vi "DAQ_E_mIO_DIO.read word.vi"(0 "i ref in":refnum<vi>, 2 "wordIndex":u32, 3 "ms timeout (10000)":i32=10000, 5 "error in (no error)":errorcluster) -> (14 "i ref out":refnum<vi>, 16 "word":u8, 17 "timed out":bool, 19 "error out":errorcluster)   [LabVIEW 2014, in "DAQ_E_mIO_DIO.lvlib"]
doc: "Reads a word from the digital input\n\nLicense Agreement for this software:\n\nCopyright (C)\nGesellschaft für Schwerionenforschung, GSI\nPlanckstr. 1\n64291 Darmstadt\nGermany\n\nContact: D.Beck@gsi.de \n\nThis program is free software; you can redistribute it and/or modify it under the terms of the GNU General Public License as published by the Free Software Foundation; either version 2 of the license, or (at your option) any later version.\n\nThis program is distributed in the hope that it will be useful, but WITHOUT ANY WARRANTY; without even the implied warranty of MERCHANTABILITY or FITNESS FOR A PARTICULAR PURPOSE. See the GNU General License for more details (http://www.gnu.org).\n\nGesellschaft für Schwerionenforschung, GSI\nPlanckstr. 1, 64291 Darmstadt, Germany\nFor all questions and ideas contact: M.Richter@gsi.de, H.Brand@gsi.de or D.Beck@gsi.de.\nLast update: 17-JUN-2004"
uses:
  DAQ_E_mIO_DIO.lvlib
  CS_Core/CSSystem/CoreDefs/CoreDefs.error_type.ctl
  CS_Core/CSApplicationBaseClasses/DigiIOBase/DigiIOBase.directionType.ctl
  CS_Core/CSApplicationBaseClasses/DigiIOBase/DigiIOBase.serviceType.ctl
  CSlibraries/UtilityLib/UtilityLib.valueStatus.ctl
  <vilib>/DAQmx/read.llb/DAQmx Read (Digital 1D Bool 1Chan 1Samp).vi
  CS_Core/CSSystem/CoreLib/CoreLib.lvlib
  CS_Core/CSApplicationBaseClasses/DigiIOBase/DigiIOBase.lvlib
  CSlibraries/UtilityLib/UtilityLib.lvlib
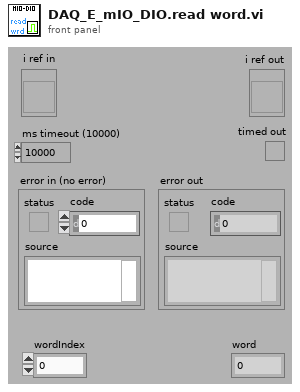
[diagram p1: front panel]
types:
  T1 = typedef "CoreDefs.error_type.ctl" = enum16{"no error", "can't load process", "can't unload process", "process does not exist", "can't install process", "can't remove process", "unknown function", "time out", "can't execute function", "duplicate queue name", "super not found", "caller queue invalid", "can't ping process", "unknown error", "VISA Error", "VISA timeout", "GPIB timeout", "GPIB error", "communication error", "data type mismatch", "can't read data from OPC server", "can't write data to OPC server", "OET error", "function not implemented", "process already exists", "invalid Shared Variable name", "error writing Shared Variable", "error reading Shared Variable", "invalid client name", "corrupt database", "unknown class", "call not authorized", "parameter out of range", "OET timeout: can't get data to modify", "invalid queue name", "requested operation incompatible with current state", "event undefined", "event disabled", "state undefined", "caller is not a friend", "EventBuilder: bad eventID", "EventBuilder: no DAQ devices", "a thread must not stop itself", "UNUSED ELEMENT4", "DiscArchiver: eventData incomplete", "DiscArchiver: eventData does not belong to run", "DiscArchiver: can't open file", "DiscArchiver: can't write to file", "DiscArchiver: available disc space low", "can't acquire semaphore", "error reading data from database", "notifier object is not existing", "can't register process", "can't unregister process", "illegal event type", "object disabled", "object already exists", "can't change state", "Instrument not found", "no connection to remote node", "invalid reference", "N/A", "UNUSED ELEMENT 1", "element not found", "illegal TCP/IP connection detected", "object does not exist", "invalid access ID", "unknown CS system", "invalid privilige", "unsupported data type", "unsupported server type", "IO server already exists", "Shared Variable already exists"}
  T2 = typedef "UtilityLib.lvlib/UtilityLib.valueStatus.ctl" = enum16{"no info available", "stand by/off", "on", "warning", "alarm/malfunction", "not implemented", "user action required", "important information", "system default", "control default", "indicator default", "button default"}
  T3 = typedef "DigiIOBase.lvlib/DigiIOBase.serviceType.ctl" = enum16{"bit", "word"}
  T4 = typedef "DigiIOBase.lvlib/DigiIOBase.directionType.ctl" = enum16{"unknown", "update actual value", "update nominal value", "update both"}
  T5 = typedef "DAQ_E_mIO_DIO.lvlib/DAQ_E_mIO_DIO.i attribute.ctl" = cluster{"DOutChannel":refnum<k21>, "DInChannel":refnum<k21>, "nOfBitsIn":i32, "nOfBitsOut":i32}
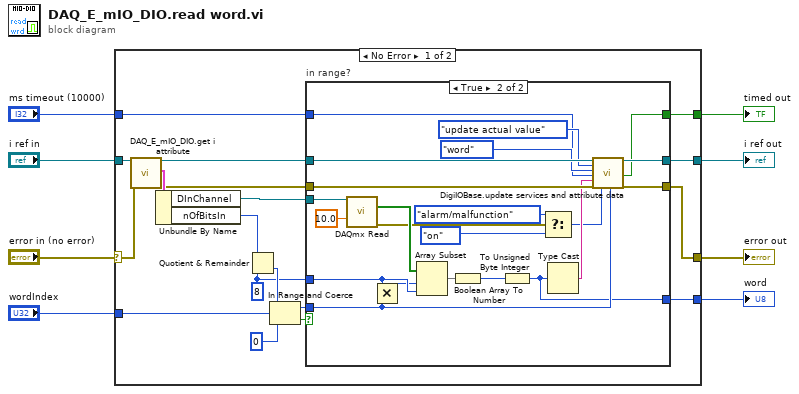
[diagram p0: block diagram]
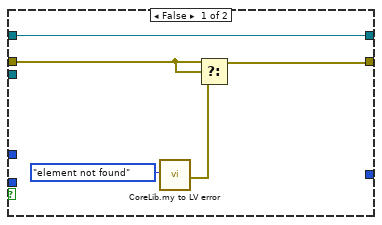
[diagram p2: hidden frame]
diagram:
  n1 = case shown="No Error" "error in (no error)" {
    selector: "error in (no error)" -> [w18 w54]
    tunnel: "i ref in" -> [w19 w55]
    tunnel: [w26 w55] -> w7
    tunnel: [w25 w54] -> w6
    tunnel: "wordIndex" -> [w23 _]
    tunnel: [w20 _] -> w4
    tunnel: "ms timeout (10000)" -> [w13 _]
    tunnel: [w12 _] -> w1
    frame No Error {
      w9 = 8 ("y")
      n2 = call "DAQ_E_mIO_DIO.get i attribute.vi"("i ref in"=w19, "error in (no error)"=w18) -> ("i ref out"=w15:refnum<vi>, "i attribute"=w17:T5, "error out"=w16:errorcluster)  [unwired: 15 in]
      n3 = Unbundle By Name(w17) -> ("DInChannel"=w14:refnum<k21>, "nOfBitsIn"=w11:i32)
      n4 = Quotient & Remainder(x=w11, y=w9) -> (floor(x/y)=w10:i32)  [unwired: 1 out]
      n5 = In Range and Coerce(upper limit=w10, x=w23, lower limit=u32 0) -> (coerced(x)=w22:u32, In Range?=w21:bool)
      n6 = case "in range?" shown="True" w21 {
        tunnel: w15 -> [w31 w50]
        tunnel: w16 -> [w30 w48]
        tunnel: [w31 w49] -> w26
        tunnel: [w29 w47] -> w25
        tunnel: w22 -> [_ w35]
        tunnel: [_ w32] -> w20
        tunnel: w14 -> [_ w52]
        tunnel: w13 -> [_ w44]
        tunnel: [_ w41] -> w12
        tunnel: w9 -> [_ w36]
        frame False {
          n7 = call "CoreLib.my to LV error.vi"("ErrorTypes"=CoreDefs.error_type."element not found") -> ("myErrorCluster"=w28:errorcluster)  [unwired: 17 in, 1 out]
          n8 = Select(t=w30, s=w30, f=w28) -> (s? t:f=w29:errorcluster)
        }
        frame True {
          n9 = call-poly <vilib>:"DAQmx Read.vi"("task/channels in"=w52, "timeout"=10.0) -> ("data"=w51:bool[], "error out"=w40:errorcluster)  [unwired: 11 in, 1 out]
          n10 = Multiply(x=w36, y=w35) -> (x*y=w34:u32)
          n11 = Array Subset(array=w51, index=w34, length=w36) -> (w43:bool[])
          n12 = Boolean Array To Number(Boolean array=w43) -> (number=w33:u32)
          n13 = To Unsigned Byte Integer(number=w33) -> (unsigned 8bit integer=w32:u8)
          n14 = Select(t=UtilityLib.valueStatus."alarm/malfunction", s=w40, f=UtilityLib.valueStatus."on" ("quality")) -> (s? t:f=w37:T2)
          n15 = Type Cast(x=w32) -> (*(type *) &x=w42:string)  [unwired: 1 in]
          n16 = call "DigiIOBase.update services and attribute data.vi"("i ref in"=w50, "direction"=DigiIOBase.directionType."update actual value", "service"=DigiIOBase.serviceType."word", "ms timeout (10000)"=w44, "value"=w42, "error in (no error)"=w48, "quality"=w37, "index"=w35) -> ("i ref out"=w49:refnum<vi>, "timed out"=w41:bool, "error out"=w47:errorcluster)  [unwired: 9 in]
        }
      }
    }
    frame Error {
    }
  }
  "error out" <- w6
  "i ref out" <- w7
  "word" <- w4
  "timed out" <- w1
